vi "toggle.vi"(1 "Input":bool) -> (0 "Output":bool)   [LabVIEW 2014]
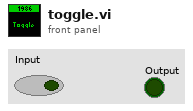
[diagram p1: front panel]
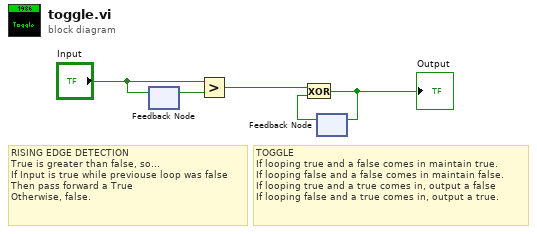
[diagram p0: block diagram]
diagram:
  # "TOGGLE\nIf looping true and a false comes in maintain true.\nIf looping false and a false comes in maintain false.\nIf looping true and a true comes in, output a false\nIf looping false and a true comes in, output a true."
  # "RISING EDGE DETECTION\nTrue is greater than false, so...\nIf Input is true while previouse loop was false\nThen pass forward a True\nOtherwise, false."
  n1 = feedback #1() -> (w1:bool)  [unwired: 1 in]
  n2 = feedback-in #1("Input") -> ()
  n3 = Greater?(x="Input", y=w1) -> (0:w3:bool)
  n4 = feedback #2() -> (w4:bool)  [unwired: 1 in]
  n5 = Exclusive Or(1:w4, 2:w3) -> (0:w5:bool)
  "Output" <- w5
  n6 = feedback-in #2(w5) -> ()
